vi "Excel Write Value.vi"(7 "reference":refnum<k7>, 8 "Value2":variant, 10 "Row":i32=1, 11 "Column":i32=1) -> (6 "reference out":refnum<k7>)   [LabVIEW 2016, in "excel.lvlib"]
uses:
  excel.lvlib
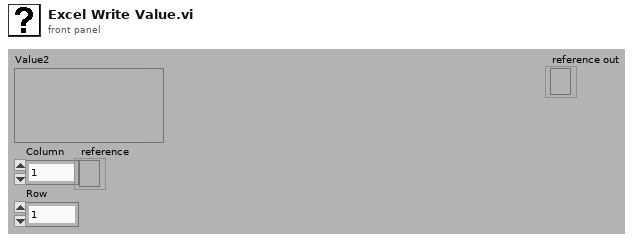
[diagram p1: front panel]
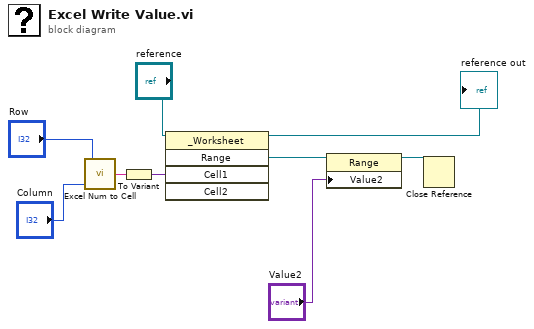
[diagram p0: block diagram]
diagram:
  n1 = call "Excel Num to Cell.vi"("Column"="Column", "Row"="Row") -> ("Cell"=w6:string)  [unwired: 3 in]
  n2 = To Variant(anything=w6) -> (Variant=w5:variant)
  n3 = invoke class="_Worksheet" method="Range"(reference="reference", "Cell1"=w5) -> (reference out=→"reference out":refnum<k7>, "Range"=w7:refnum<k7>)  [unwired: 3 in, 3 out]
  n4 = property class="Range"(reference=w7, "Value2"="Value2") -> (reference out=w1:refnum<k7>)  [unwired: 1 in, 1 out]
  n5 = Close Reference(reference=w1) -> ()  [unwired: 1 in, 1 out]
